vi "pump to booleans.vi"(1 "Control":T1={"Switches"=[FALSE, FALSE, FALSE, FALSE, FALSE, FALSE, FALSE, FALSE, FALSE, FALSE, FALSE, FALSE, FALSE], "Pumps"=[{"on/off"=FALSE, "Direction"=FALSE, "flow rate"=0.0, "Tubing"=enum."orange-black", "tubing or 0 to 1"=FALSE, "0 to 1"=0.0}, {"on/off"=FALSE, "Direction"=FALSE, "flow rate"=0.0, "Tubing"=enum."orange-black", "tubing or 0 to 1"=FALSE, "0 to 1"=0.0}, {"on/off"=FALSE, "Direction"=FALSE, "flow rate"=0.0, "Tubing"=enum."orange-black", "tubing or 0 to 1"=FALSE, "0 to 1"=0.0}, {"on/off"=FALSE, "Direction"=FALSE, "flow rate"=0.0, "Tubing"=enum."orange-black", "tubing or 0 to 1"=FALSE, "0 to 1"=0.0}, {"on/off"=FALSE, "Direction"=FALSE, "flow rate"=0.0, "Tubing"=enum."orange-black", "tubing or 0 to 1"=FALSE, "0 to 1"=0.0}, {"on/off"=FALSE, "Direction"=FALSE, "flow rate"=0.0, "Tubing"=enum."orange-black", "tubing or 0 to 1"=FALSE, "0 to 1"=0.0}]} {"Pumps"."0 to 1" format="%.2f"; "Pumps"."flow rate" format="%.2f"}) -> (0 "controls boolean":bool[](array[boolean]))   [LabVIEW 2015]
uses:
  Stamp 2 control.ctl
  Peristaltic/Pump w direction.ctl
  mini peristaltic pump.ctl
  Pump Direction.ctl
  3-stop colors and numbers.ctl
panel:
  # "0-12"
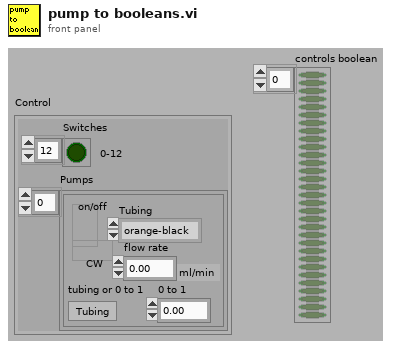
[diagram p1: front panel]
types:
  T1 = typedef "Stamp 2 control.ctl" = cluster{"Switches":bool[], "Pumps":T2[]}
  T2 = typedef "Pump w direction.ctl" = cluster{"on/off":T3, "Direction":T4, "flow rate":dbl[unit], "Tubing":T5, "tubing or 0 to 1":bool, "0 to 1":dbl}
  T3 = typedef "mini peristaltic pump.ctl" = bool
  T4 = typedef "Pump Direction.ctl" = bool
  T5 = typedef "3-stop colors and numbers.ctl" = enum16{"orange-black", "orange-red", "orange-blue", "orange-green", "green-yellow", "orange-yellow", "white-yellow", "orange-white", "black-black", "orange-orange", "white-black", "white-white", "white-red", "red-red", "red-grey", "grey-grey", "yellow-yellow", "yellow-blue", "blue-blue", "blue-green", "green-green", "purple-purple", "purple-black", "purple-orange", "purple-white", "black-white", "13", "14", "15", "16", "17", "18"}
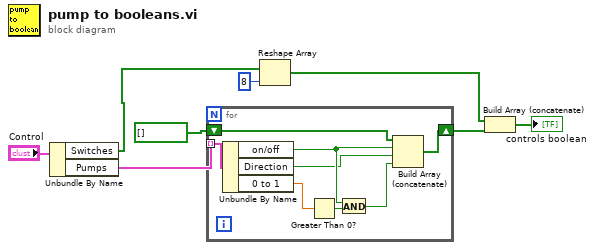
[diagram p0: block diagram]
diagram:
  n1 = Unbundle By Name("Control") -> ("Switches"=w5:bool[], "Pumps"=w7:T2[])
  n2 = for {
    tunnel: w7 -> [w16] mode=indexing
    shift-right: [w10] -> w4
    shift-left: bool[] [] -> [w9]
    n3 = Unbundle By Name(w16) -> ("on/off"=w13:T3, "Direction"=w12:T4, "0 to 1"=w15:dbl)
    n4 = Greater Than 0?(x=w15) -> (x > 0?=w14:bool)
    n5 = And(x=w13, y=w14) -> (x .and. y?=w11:T3)
    n6 = Build Array (concatenate)(w9, w13, w12, w11) -> (w10:T3[])
  }
  n7 = Reshape Array(w5, 8 ("dimension size")) -> (w2:bool[])
  n8 = Build Array (concatenate)(w2, w4) -> (→"controls boolean":T3[])
